vi "Insert VI Index.vi"(6 "Size":T2, 7 "Position":T1, 8 "error in (no error)":errorcluster, 9 "Z-Order":i32, 10 "VI Refnum":refnum<vi>, 11 "WindowFrame in":refnum<class "WindowFrame.lvclass">) -> (0 "error out":errorcluster, 3 "WindowFrame out":refnum<class "WindowFrame.lvclass">)   [LabVIEW 2021, in "WindowFrame.lvlib" / "WindowFrame.lvclass"]
uses:
  WindowFrame.lvclass
  <vilib>/Utility/miscctls.llb/LVBoundsTypeDef.ctl
  <vilib>/Utility/miscctls.llb/LVPositionTypeDef.ctl
  SubPanelInfo.ctl
  Action.ctl
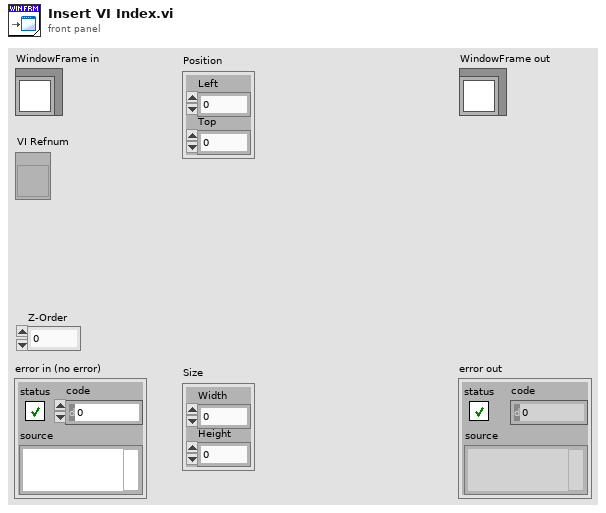
[diagram p1: front panel]
types:
  T1 = typedef "LVPositionTypeDef.ctl" = cluster{"Left":i32, "Top":i32}
  T2 = typedef "LVBoundsTypeDef.ctl" = cluster{"Width":u32, "Height":u32}
  T3 = typedef "WindowFrame.lvlib/WindowFrame.lvclass/SubPanelInfo.ctl" = cluster{"Z-Order":i32, "Position":T1, "Size":T2, "VI Ref":refnum<vi>}
  T4 = typedef "WindowFrame.lvlib/WindowFrame.lvclass/Action.ctl" = enum16{"Set Allow Runtime PopUp", "Set Behavior", "Set Closable", "Set Custom Title", "Set Highlight Return Button", "Set Is Frontmost", "Set Minimizable", "Set Minimum Size", "Set Monitor", "Set Resizable", "Set Panel Bounds", "Set Run VI Transparently", "Set Show Menu Bar", "Set State", "Set Title", "Set Title Bar Colors", "Set Title Bar Visible", "Set Transparancy", "Set Window Bounds", "Get Allow Runtime PopUp", "Get Behavior", "Get Closable", "Get Custom Title", "Get Highlight Return Button", "Get Is Frontmost", "Get Minimizable", "Get Minimum Size", "Get Monitor", "Get Panel Bounds", "Get Resizable", "Get Run VI Transparently", "Get Show Menu Bar", "Get State", "Get Title", "Get Title Bar Colors", "Get Title Bar Visible", "Get Transparancy", "Get Window Bounds", "--", "Center", "Close", "Open", "Run-Time Position:Centered", "Run-Time Position:Custom", "Run-Time Position:Get Position", "Run-Time Position:Maximized", "Run-Time Position:Minimized", "Run-Time Position:Unchanged", "---", "Insert VI", "Remove VI", "Insert VI Index", "Remove VI Index", "Exit"}
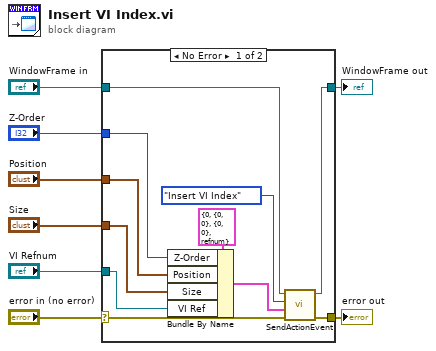
[diagram p0: block diagram]
diagram:
  n1 = case shown="No Error" "error in (no error)" {
    selector: "error in (no error)" -> [w15 w21]
    tunnel: [w19 w21] -> w7
    tunnel: [w17 w20] -> w5
    tunnel: "WindowFrame in" -> [w16 w20]
    tunnel: "VI Refnum" -> [w9 _]
    tunnel: "Z-Order" -> [w12 _]
    tunnel: "Position" -> [w11 _]
    tunnel: "Size" -> [w10 _]
    frame No Error {
      n2 = Bundle By Name(cluster=T3 {"Z-Order"=0, "Position"={"Left"=0, "Top"=0}, "Size"={"Width"=0, "Height"=0}, "VI Ref"=refnum} ("Cluster"), "Z-Order"=w12, "Position"=w11, "Size"=w10, "VI Ref"=w9) -> (w13:T3)
      n3 = call "SendActionEvent.vi"("error in (no error)"=w15, "Variant"=w13, "Action"=Action."Insert VI Index", "WindowFrame in"=w16) -> ("error out"=w19:errorcluster, "WindowFrame out"=w17:refnum<class "WindowFrame.lvclass">)  [unwired: 6 in]
    }
    frame Error {
    }
  }
  "error out" <- w7
  "WindowFrame out" <- w5
